vi "Rectangle Comparison.vi"(8 "Angle (deg)":dbl, 9 "Second":dbl[](array[numeric]), 11 "First":dbl[](array[numeric])) -> (0 "Rect":T1, 3 "Scores":T2)   [LabVIEW 2025]
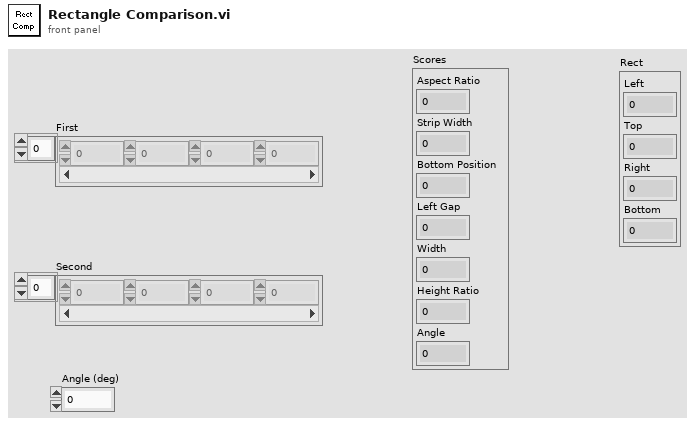
[diagram p1: front panel]
types:
  T1 = cluster{"Left":dbl, "Top":dbl, "Right":dbl, "Bottom":dbl}
  T2 = cluster{"Aspect Ratio":dbl, "Strip Width":dbl, "Bottom Position":dbl, "Left Gap":dbl, "Width":dbl, "Height Ratio":dbl, "Angle":dbl}
  T3 = cluster{"[0]":dbl, "[1]":dbl, "[2]":dbl, "[3]":dbl}
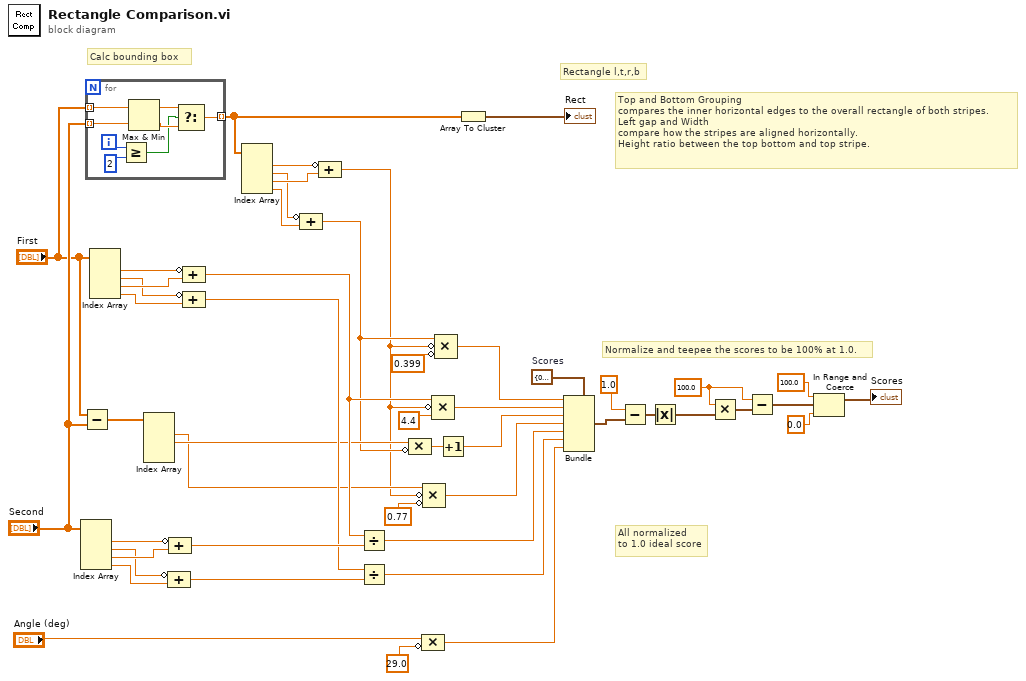
[diagram p0: block diagram]
diagram:
  w1 = T2 {"Aspect Ratio"=0.0, "Strip Width"=0.0, "Bottom Position"=0.0, "Left Gap"=0.0, "Width"=0.0, "Height Ratio"=0.0, "Angle"=0.0}  # Scores
  w36 = 100.0 ("x/y")
  # "All normalized\nto 1.0 ideal score"
  # "Normalize and teepee the scores to be 100% at 1.0."
  # "Top and Bottom Grouping\ncompares the inner horizontal edges to the overall rectangle of both stripes.\nLeft gap and Width\ncompare how the stripes are aligned horizontally.\nHeight ratio between the top bottom and top stripe."
  # "Calc bounding box"
  # "Rectangle l,t,r,b"
  n1 = Index Array(array="Second") -> (element #1=w46:dbl, element #2=w27:dbl, element #3=w49:dbl, element #4=w11:dbl)  [unwired: 4 in]
  n2 = Subtract(x="First", y="Second") -> (x-y=w18:dbl[])
  n3 = for {
    tunnel: "First" -> [w57] mode=indexing
    tunnel: "Second" -> [w56] mode=indexing
    tunnel: [w50] -> w21 mode=indexing
    i -> [w54]
    n4 = Greater Or Equal?(x=w54, y=2) -> (x >= y?=w51:bool)
    n5 = Max & Min(x=w57, y=w56) -> (max(x,y)=w53:dbl, min(x,y)=w52:dbl)
    n6 = Select(t=w53, s=w51, f=w52) -> (s? t:f=w50:dbl)
  }
  n7 = Index Array(array="First") -> (element #1=w41:dbl, element #2=w26:dbl, element #3=w40:dbl, element #4=w42:dbl)  [unwired: 4 in]
  n8 = Index Array(array=w18) -> (element #1=w16:dbl, element #2=w17:dbl)  [unwired: 4 in, 2 out]
  n9 = Compound Arithmetic op=ADD(invert w27, w11) -> (w47:dbl)
  n10 = Compound Arithmetic op=ADD(invert w46, w49) -> (w48:dbl)
  n11 = Compound Arithmetic op=ADD(invert w41, w40) -> (w24:dbl)
  n12 = Compound Arithmetic op=ADD(invert w26, w42) -> (w28:dbl)
  n13 = Index Array(array=w21) -> (element #1=w13:dbl, element #2=w10:dbl, element #3=w12:dbl, element #4=w9:dbl)  [unwired: 4 in]
  n14 = Compound Arithmetic op=ADD(invert w10, w9) -> (w8:dbl)
  n15 = Compound Arithmetic op=ADD(invert w13, w12) -> (w7:dbl)
  n16 = Divide(x=w24, y=w48) -> (x/y=w44:dbl)
  n17 = Divide(x=w28, y=w47) -> (x/y=w43:dbl)
  n18 = Compound Arithmetic op=MULTIPLY(w17, invert w8) -> (w23:dbl)
  n19 = Compound Arithmetic op=MULTIPLY("Angle (deg)", invert 29.0 ("y")) -> (w2:dbl)
  n20 = Compound Arithmetic op=MULTIPLY(w16, invert w7, invert 0.77 ("y")) -> (w19:dbl)
  n21 = Compound Arithmetic op=MULTIPLY(w24, invert w7, 4.4 ("y")) -> (w45:dbl)
  n22 = Compound Arithmetic op=MULTIPLY(w8, invert w7, invert 0.399 ("y")) -> (w5:dbl)
  n23 = Increment(x=w23) -> (x+1=w22:dbl)
  n24 = Array To Cluster(array=w21) -> (cluster=→"Rect":T3)
  n25 = Bundle(cluster=w1, "Aspect Ratio"=w5, "Strip Width"=w45, "Bottom Position"=w22, "Left Gap"=w19, "Width"=w44, "Height Ratio"=w43, "Angle"=w2) -> (w30:T2)
  n26 = Subtract(x=1.0 ("y"), y=w30) -> (x-y=w34:T2)
  n27 = Absolute Value(x=w34) -> (abs(x)=w37:T2)
  n28 = Multiply(x=w36, y=w37) -> (x*y=w38:T2)
  n29 = Subtract(x=w36, y=w38) -> (x-y=w33:T2)
  n30 = In Range and Coerce(upper limit=100.0, x=w33, lower limit=0.0) -> (coerced(x)=→"Scores":T2)  [unwired: 1 out]
